vi "Oscop Read.vi"(7 "Perform Auto Setup":bool, 8 "error in (no error)":errorcluster, 9 "Measurement (0: Vpp)":u16(ring) items=["Vpp", "Vmax", "Vmin", "Vamp", "Vtop", "Vbase", "Vavg", "Mean", "Vrms", "Crms", "FOV", "FPRE", "ROV", "RPRE", "Period", "Freq", "+Wid", "-Wid", "Rise Time", "Fall Time", "Bwid", "+Duty", "-Duty"], 10 "Source (1: Channel 1)":u16(ring)=1 items=["Channel 1"=1, "Channel 2"=2, "Channel 3"=3, "Channel 4"=4], 11 "VISA resource name":refnum<visa-resource-name>) -> (0 "error out":errorcluster, 2 "Value":dbl, 3 "VISA resource name out":refnum<visa-resource-name>)   [LabVIEW 2021]
uses:
  Program Files/National Instruments/LabVIEW 2021/instr.lib/Siglent SDS 1000 2000 Series/Public/Data/Read Waveform Measurement (Standard).vi
  Program Files/National Instruments/LabVIEW 2021/instr.lib/Siglent SDS 1000 2000 Series/Siglent SDS 1000 2000 Series.lvlib
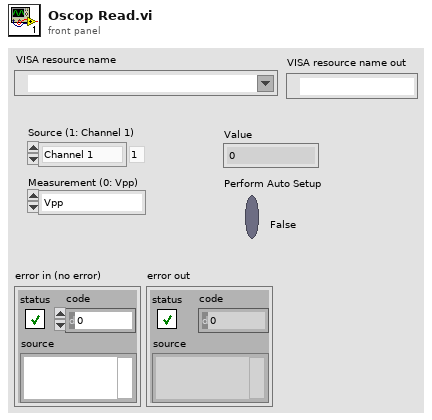
[diagram p1: front panel]
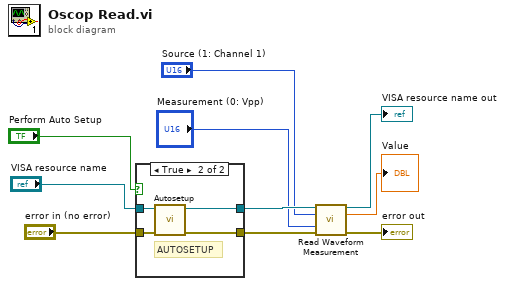
[diagram p0: block diagram]
diagram:
  n1 = case shown="True" "Perform Auto Setup" {
    tunnel: "error in (no error)" -> [w11 w16]
    tunnel: "VISA resource name" -> [w12 w15]
    tunnel: [w12 w14] -> w9
    tunnel: [w11 w13] -> w8
    frame False {
    }
    frame True {
      # "AUTOSETUP"
      n2 = call "Autosetup.vi"("error in (no error)"=w16, "VISA resource name"=w15) -> ("error out"=w13:errorcluster, "VISA resource name out"=w14:refnum<visa-resource-name>)  [unwired: 8 in]
    }
  }
  n3 = call-poly "Read Waveform Measurement.vi"("VISA resource name"=w9, "Source (1: Channel 1)"="Source (1: Channel 1)", "Measurement (0: Vpp)"="Measurement (0: Vpp)", "error in (no error)"=w8) -> ("VISA resource name out"=→"VISA resource name out":refnum<visa-resource-name>, "Value"=→"Value":dbl, "error out"=→"error out":errorcluster)  [unwired: 9 in]
